vi "ROI entry-ROI tools management.vi"(7 "Initialise":bool, 8 "error in (no error)":errorcluster, 11 "ROI Enum":T1) -> (0 "error out":errorcluster)   [LabVIEW 2020]
uses:
  Typedefs/ROI ID Enum.ctl
  Globals/gl_ROI Entry UI globals.vi
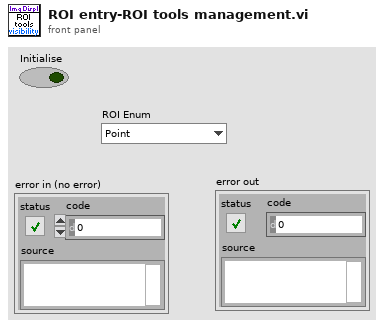
[diagram p1: front panel]
types:
  T1 = typedef "ROI ID Enum.ctl" = enum16{"Point", "MiniScan", "Comp. MiniScan", "Rectangle", "Comp. volume", "Arb. plane point", "None"}
  T2 = typedef "ROI entry screen ctrl refs cluster.ctl" = cluster{"Done button":refnum<vi>, "Imaging button":refnum<vi>, "Acquisition button":refnum<vi>, "Scan dwell time per pixel (us)":refnum<vi>, "# of planes":refnum<vi>, "Zoom Ctrl":refnum<vi>, "Equal size":refnum<vi>, "Channel":refnum<vi>, "Image Display":refnum<vi>, "Z-Plane Selector":refnum<vi>, "Number of lines left":refnum<vi>, "Z-stack folder path":refnum<vi>, "POI Density":refnum<vi>, "Arb Plane Entry":refnum<vi>, "Whole Plane":refnum<vi>, "Line Mode":refnum<vi>, "Clear Last":refnum<vi>, "Clear All":refnum<vi>, "Delete Lines":refnum<vi>, "Trial Length (sec)":refnum<vi>, "Palette Type":refnum<vi>, "Intensity slider":refnum<vi>, "# POI":refnum<vi>, "Max Z Proj":refnum<vi>, "Zplane ind":refnum<vi>, "Wavelength (nm)":refnum<vi>, "Number of Trials":refnum<vi>, "Funct stim.trig.enable":refnum<vi>, "Funct stim.trig.delay (s)":refnum<vi>, "Line Mode":refnum<vi>, "Step size (µm)":refnum<vi>, "ROI move mode":refnum<vi>, "Cool-down time (s)":refnum<vi>, "Enable cool-down time":refnum<vi>, "Motor Z ind. (um)":refnum<vi>, "AOL Z ind. (um)":refnum<vi>, "Load Reference Image":refnum<vi>, "Rel.  Res.":refnum<vi>, "ROI LIST":refnum<vi>, "Show All":refnum<vi>, "ROI Type":refnum<vi>, "Start Plane":refnum<vi>, "Stop Plane":refnum<vi>, "Offset ROI":refnum<vi>, "Tab Control":refnum<vi>, "Laser Power(%)":refnum<vi>, "Cycle rate":refnum<vi>, "FOV (Ind.)":refnum<vi>, "Frame Size (Ind.)":refnum<vi>, "Resolution (Ind.)":refnum<vi>, "Pixel Density (Ind)":refnum<vi>, "Laser Power (Ind.)":refnum<vi>, "Dwell Time (Ind.)":refnum<vi>, "Adj MC":refnum<vi>}
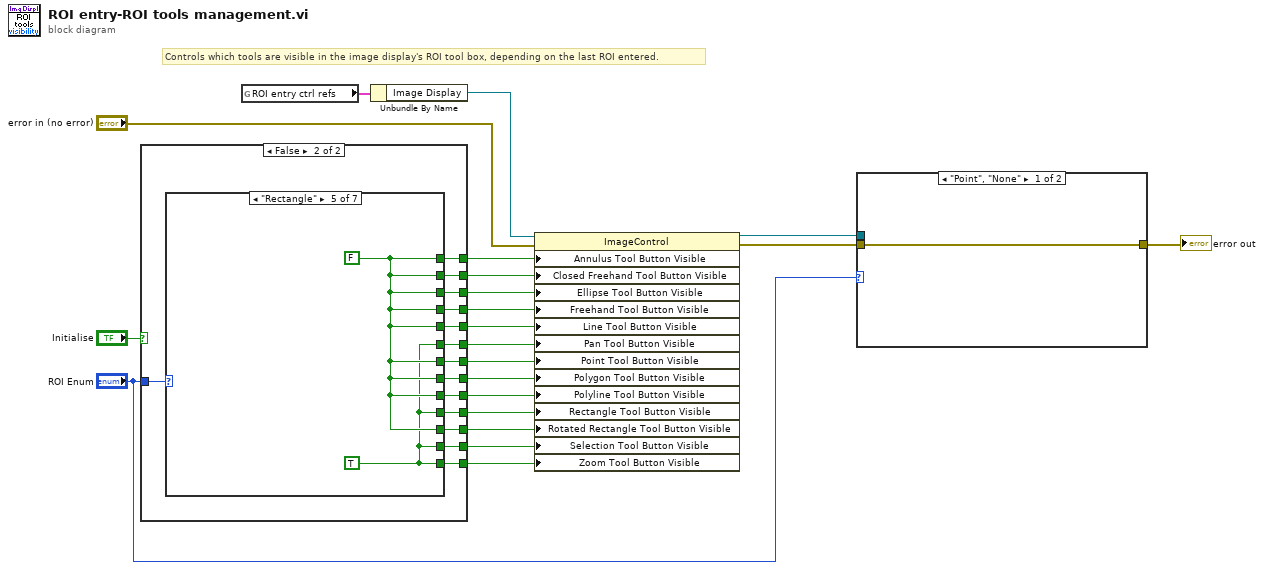
[diagram p0: block diagram]
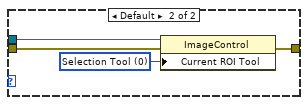
[diagram p2: hidden frame]
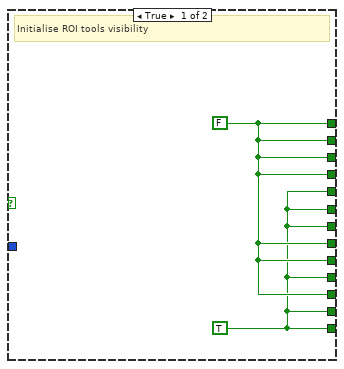
[diagram p3: hidden frame]
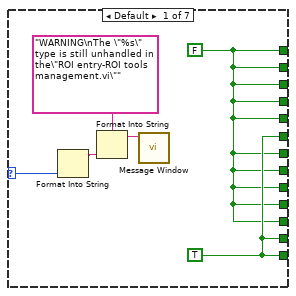
[diagram p4: hidden frame]
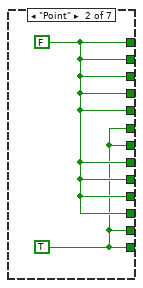
[diagram p5: hidden frame]
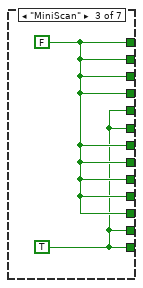
[diagram p6: hidden frame]
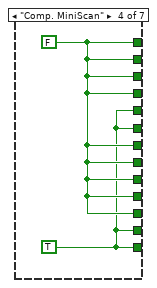
[diagram p7: hidden frame]
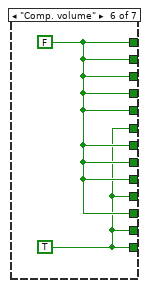
[diagram p8: hidden frame]
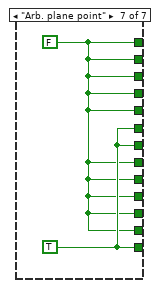
[diagram p9: hidden frame]
diagram:
  # "Controls which tools are visible in the image display's ROI tool box, depending on the last ROI entered."
  n1 = case shown="False" "Initialise" {
    tunnel: "ROI Enum" -> [_ w37]
    tunnel: [w23 w36] -> w20
    tunnel: [w23 w35] -> w19
    tunnel: [w23 w34] -> w18
    tunnel: [w23 w33] -> w17
    tunnel: [w23 w32] -> w16
    tunnel: [w23 w31] -> w15
    tunnel: [w22 w30] -> w14
    tunnel: [w23 w29] -> w13
    tunnel: [w22 w28] -> w12
    tunnel: [w22 w27] -> w11
    tunnel: [w22 w26] -> w10
    tunnel: [w22 w25] -> w9
    tunnel: [w22 w24] -> w8
    frame True {
      w22 = TRUE
      w23 = FALSE
      # "Initialise ROI tools visibility"
    }
    frame False {
      n2 = case shown="\"Rectangle\"" w37 {
        selector: w37 -> [w40 _ _ _ _ _ _]
        tunnel: [w42 w45 w47 w49 w51 w53 w54] -> w36
        tunnel: [w42 w45 w47 w49 w51 w53 w54] -> w35
        tunnel: [w42 w45 w47 w49 w51 w53 w54] -> w34
        tunnel: [w42 w45 w47 w49 w51 w53 w54] -> w33
        tunnel: [w42 w45 w47 w49 w51 w53 w54] -> w32
        tunnel: [w42 w45 w47 w49 w51 w53 w54] -> w31
        tunnel: [w42 w45 w47 w49 w50 w52 w54] -> w30
        tunnel: [w42 w45 w47 w49 w51 w53 w54] -> w29
        tunnel: [w42 w44 w47 w49 w51 w53 w55] -> w28
        tunnel: [w42 w45 w46 w48 w51 w53 w54] -> w27
        tunnel: [w43 w44 w46 w48 w50 w52 w55] -> w26
        tunnel: [w43 w44 w46 w48 w50 w52 w54] -> w25
        tunnel: [w43 w44 w46 w48 w50 w52 w55] -> w24
        frame Default {
          w43 = TRUE
          w42 = FALSE
          n3 = Format Into String(w40) -> (resulting string=w39:string)  [unwired: 3 in, 1 out]
          n4 = Format Into String(format string="WARNING\nThe \"%s\" type is still unhandled in the\"ROI entry-ROI tools management.vi\"" ("Message string"), w39) -> (resulting string=w38:string)  [unwired: 2 in, 1 out]
          n5 = call "Message Window.vi"("Message string"=w38) -> ()  [unwired: 10 in, 1 out]
        }
        frame "Point" {
          w44 = TRUE
          w45 = FALSE
        }
        frame "MiniScan" {
          w46 = TRUE
          w47 = FALSE
        }
        frame "Comp. MiniScan" {
          w48 = TRUE
          w49 = FALSE
        }
        frame "Rectangle" {
          w50 = TRUE
          w51 = FALSE
        }
        frame "Comp. volume" {
          w52 = TRUE
          w53 = FALSE
        }
        frame "Arb. plane point" {
          w55 = TRUE
          w54 = FALSE
        }
      }
    }
  }
  n6 = global read "gl_ROI Entry UI globals.vi" "ROI entry ctrl refs"() -> (w21:T2)
  n7 = Unbundle By Name(w21) -> ("Image Display"=w7:refnum<vi>)
  n8 = property class="ImageControl"(reference=w7, error in="error in (no error)", "Annulus Tool Button Visible"=w20, "Closed Freehand Tool Button Visible"=w19, "Ellipse Tool Button Visible"=w18, "Freehand Tool Button Visible"=w17, "Line Tool Button Visible"=w11, "Pan Tool Button Visible"=w10, "Point Tool Button Visible"=w12, "Polygon Tool Button Visible"=w16, "Polyline Tool Button Visible"=w15, "Rectangle Tool Button Visible"=w14, "Rotated Rectangle Tool Button Visible"=w13, "Selection Tool Button Visible"=w9, "Zoom Tool Button Visible"=w8) -> (reference out=w4:refnum<vi>, error out=w3:errorcluster)
  n9 = case shown="\"Point\", \"None\"" "ROI Enum" {
    tunnel: w4 -> [_ w60]
    tunnel: w3 -> [w56 w59]
    tunnel: [w56 w58] -> w2
    frame "Point", "None" {
    }
    frame Default {
      w57 = u32 0 items=["Zoom Tool"=8, "Selection Tool"=0, "Pan Tool"=9, "Point Tool"=1, "Line Tool"=2, "Rectangle Tool"=3, "Rotated Rectangle Tool"=12, "Polyline Tool"=10, "Polygon Tool"=5, "Freehand Tool"=11, "Closed Freehand Tool"=6, "Ellipse Tool"=4, "Annulus Tool"=7] ("Current ROI Tool")
      n10 = property class="ImageControl"(reference=w60, error in=w59, "Current ROI Tool"=w57) -> (error out=w58:errorcluster)  [unwired: 1 out]
    }
  }
  "error out" <- w2
